vi "DatatoGraphPP.vi"(0 "PacificPowerChartReference":refnum<vi>, 5 "Measurement Cluster":T1, 9 "PlotYAxis":u32[](array[numeric]), 11 "error in (no error)":errorcluster) -> (4 "Array":waveform(dbl)[](array[waveform]), 6 "Incorrect DataType?":bool, 15 "error out":errorcluster)   [LabVIEW 2018, in "AcPwrPlugins.lvlib" / "PacificPowerSource.lvclass"]
uses:
  AcPwrPlugins/PacificPowerSource/PacificPowerSource.lvclass
  AcPwrPlugins/PacificPowerSource/TypeDefs/MeasurementData.ctl
  AcPwrPlugins/PacificPowerSource/TypeDefs/Measurements.ctl
  AcPwrPlugins/PacificPowerSource/TypeDefs/MeasurementType.ctl
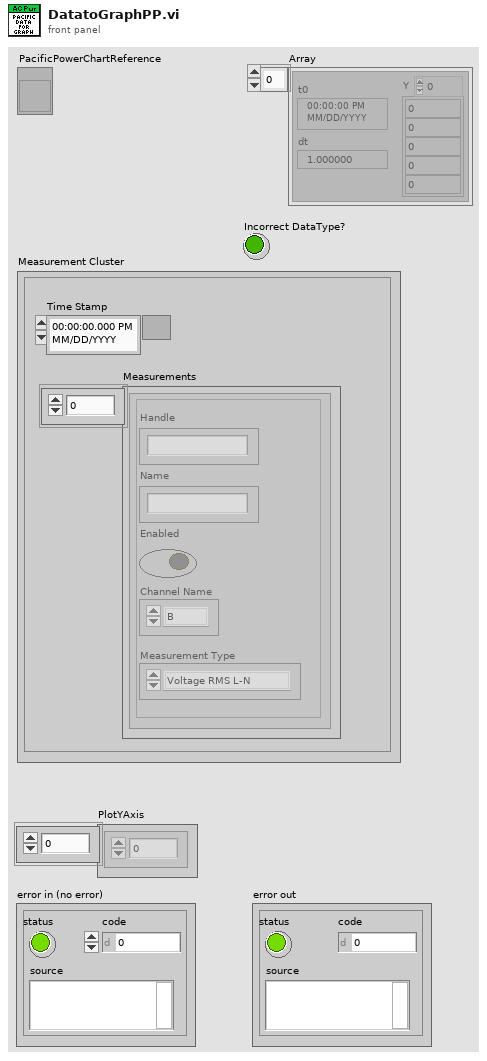
[diagram p1: front panel]
types:
  T1 = typedef "AcPwrPlugins.lvlib/PacificPowerSource.lvclass/MeasurementData.ctl" = cluster{"Time Stamp":timestamp, "Measurements":T2}
  T2 = typedef "AcPwrPlugins.lvlib/PacificPowerSource.lvclass/Measurements.ctl" = cluster{"Handle":string, "Name":string, "Enabled ":bool, "Measurement Value":dbl, "Channel Name":enum16{"A", "B", "C"}, "Measurement Type ":T3}[]
  T3 = typedef "AcPwrPlugins.lvlib/PacificPowerSource.lvclass/MeasurementType.ctl" = enum16{"Voltage RMS L-N", "Voltage RMS L-L", "Frequency", "Current RMS", "Current Peak", "Crest Factor", "Power Factor", "Power VA", "Real Power"}
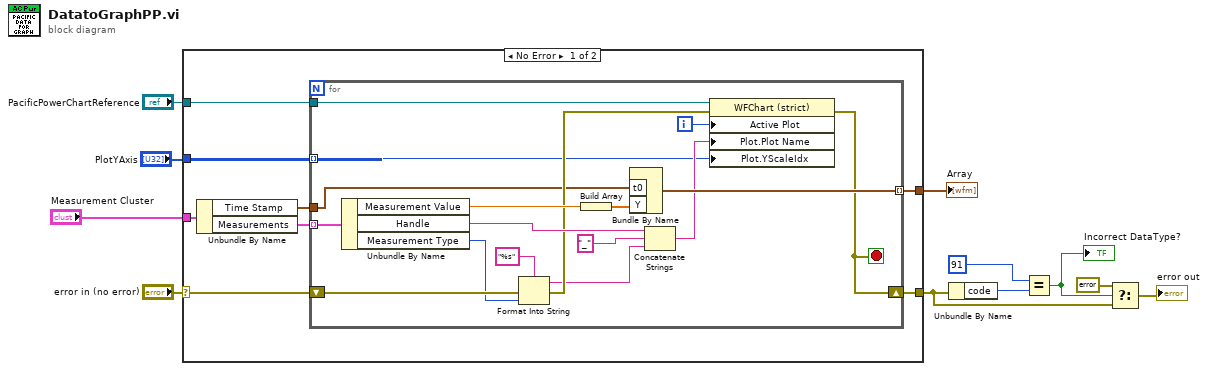
[diagram p0: block diagram]
diagram:
  n1 = case shown="No Error" "error in (no error)" {
    selector: "error in (no error)" -> [w15 w37]
    tunnel: [w19 _] -> w4
    tunnel: "Measurement Cluster" -> [w14 _]
    tunnel: [w18 w37] -> w5
    tunnel: "PacificPowerChartReference" -> [w16 _]
    tunnel: "PlotYAxis" -> [w17 _]
    frame No Error {
      n2 = Unbundle By Name(w14) -> ("Time Stamp"=w12:timestamp, "Measurements"=w13:T2)
      n3 = for {
        shift-right: [w23] -> w18
        shift-left: w15 -> [w26]
        tunnel: [w36] -> w19 mode=indexing
        tunnel: w16 -> [w25]
        tunnel: w17 -> [w24] mode=indexing
        tunnel: w13 -> [w20] mode=indexing
        tunnel: w12 -> [w21]
        i -> [w35]
        stop <- w23 stop-if-true
        n4 = Unbundle By Name(w20) -> ("Measurement Value"=w34:dbl, "Handle"=w32:string, "Measurement Type"=w22:T3)
        n5 = Format Into String(format string="%s", error in=w26, w22) -> (resulting string=w29:string, error out=w30:errorcluster)  [unwired: 1 in]
        n6 = Build Array(w34) -> (w33:dbl[])
        n7 = Bundle By Name("t0"=w21, "Y"=w33) -> (w36:waveform(dbl))  [unwired: 1 in]
        n8 = Concatenate Strings(w32, "_" ("string"), w29) -> (w28:string)
        n9 = property on="Property Node" class="WFChart (strict)"(reference=w25, error in=w30, "Active Plot"=w35, "Plot.Plot Name"=w28, "Plot.YScaleIdx"=w24) -> (error out=w23:errorcluster)  [unwired: 1 out]
      }
    }
    frame Error {
    }
  }
  "Array" <- w4
  n10 = Unbundle By Name(w5) -> ("code"=w3:i32)
  n11 = Equal?(x=91 ("y"), y=w3) -> (x = y?=w8:bool)
  "Incorrect DataType?" <- w8
  n12 = Select(t=errorcluster {"status"=FALSE, "code"=0, "source"=""} ("error IO"), s=w8, f=w5) -> (s? t:f=→"error out":errorcluster)
